vi "Number to String.vi"(8 "error in (no error)":errorcluster, 10 "desired minimum string length":i32=10 min=1 max=10, 11 "Number":i32=1445234 min=0) -> (0 "error out":errorcluster, 3 "String":string)   [LabVIEW 2019]
doc: "Converts a <b>Number</b> to a <b>String</b> of fixed length.\n\nExample: If <b>Length</b> = 6:\n5 becomes 000005\n199999 becomes 199999"
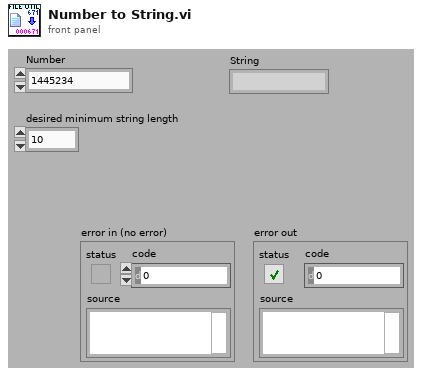
[diagram p1: front panel]
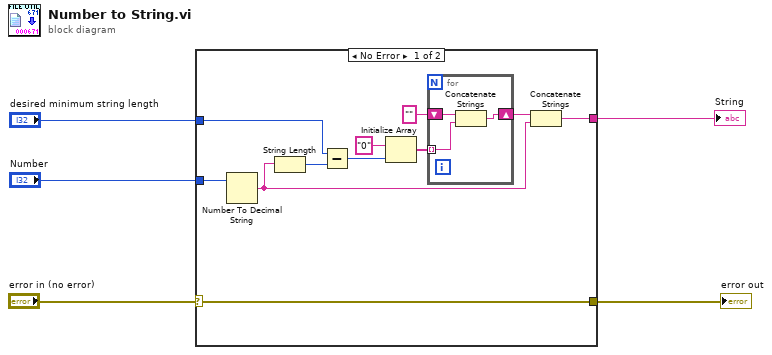
[diagram p0: block diagram]
diagram:
  n1 = case shown="No Error" "error in (no error)" {
    selector: "error in (no error)" -> [w6 w20]
    tunnel: "Number" -> [w16 _]
    tunnel: "desired minimum string length" -> [w9 _]
    tunnel: [w8 _] -> w3
    tunnel: [w6 w20] -> w1
    frame No Error {
      n2 = Number To Decimal String(number=w16) -> (decimal integer string=w15:string)  [unwired: 1 out]
      n3 = String Length(string=w15) -> (length=w10:i32)
      n4 = Subtract(x=w9, y=w10) -> (x-y=w11:i32)
      n5 = Initialize Array("0" ("string"), w11) -> (w7:string[])
      n6 = for {
        tunnel: w7 -> [w19] mode=indexing
        shift-right: [w18] -> w12
        shift-left: "" -> [w17]
        n7 = Concatenate Strings(w17, w19) -> (w18:string)
      }
      n8 = Concatenate Strings(w12, w15) -> (w8:string)
    }
    frame Error {
    }
  }
  "String" <- w3
  "error out" <- w1
